vi "Plot.vi"(4 "Response Inverted?":bool, 6 "Stimulus Inverted?":bool, 8 "error in (no error)":errorcluster, 10 "Graph Manager.lvclass":refnum<class "Graph Manager.lvclass">, 11 "Sinusoidal Fit in":refnum<class "Abstract Fit.lvclass">) -> (0 "error out":errorcluster, 1 "Channel IDs":i32[](array[numeric]), 2 "Graph Manager.lvclass 2":refnum<class "Graph Manager.lvclass">, 3 "Sinusoidal Fit out":refnum<class "Abstract Fit.lvclass">)   [LabVIEW 2016, in "Abstract Fit.lvclass"]
uses:
  Abstract Fit.lvclass
  Graph Manager/Graph Manager.lvclass
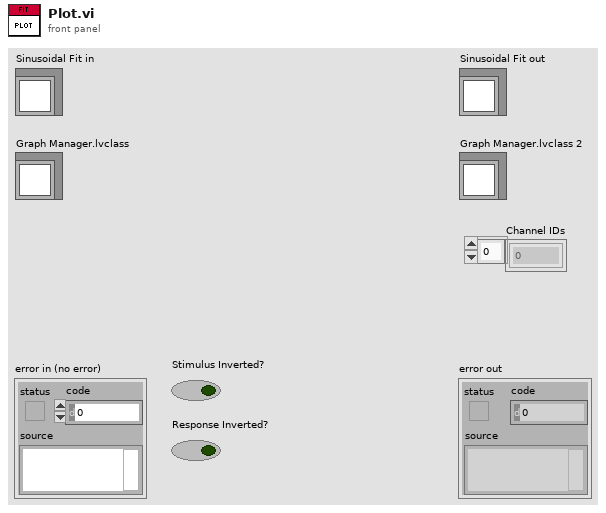
[diagram p1: front panel]
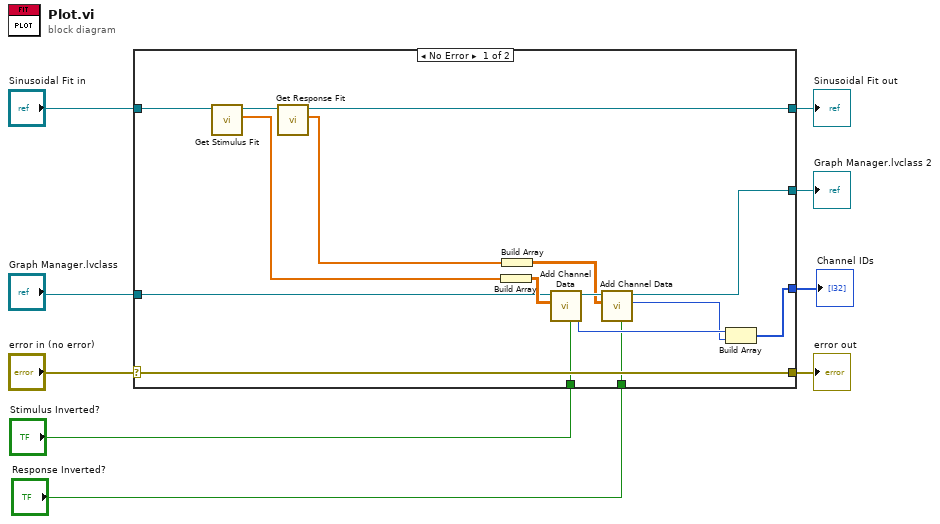
[diagram p0: block diagram]
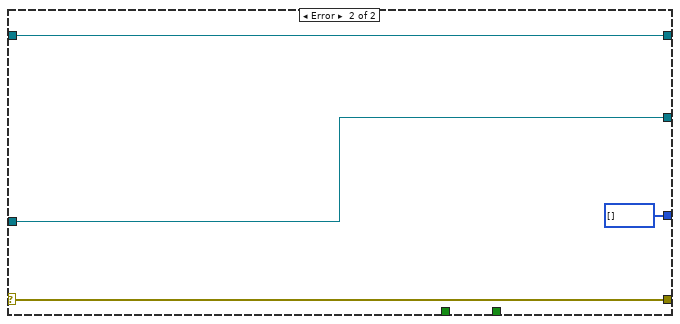
[diagram p2: hidden frame]
diagram:
  n1 = case shown="No Error" "error in (no error)" {
    selector: "error in (no error)" -> [w25 w29]
    tunnel: [w25 w29] -> w8
    tunnel: [w21 w28] -> w6
    tunnel: "Sinusoidal Fit in" -> [w23 w28]
    tunnel: "Graph Manager.lvclass" -> [w19 w27]
    tunnel: [w15 w27] -> w4
    tunnel: [w17 i32[] []] -> w3
    tunnel: "Stimulus Inverted?" -> [w11 _]
    tunnel: "Response Inverted?" -> [w10 _]
    frame No Error {
      n2 = call-dynamic "Get Stimulus Fit.vi"("Abstract Fit in"=w23) -> ("Fit out"=w20:dbl[], "Abstract Fit out"=w22:refnum<class "Abstract Fit.lvclass">)  [unwired: 8 in, 1 out]
      n3 = call-dynamic "Get Response Fit.vi"("Abstract Fit in"=w22) -> ("Fit out"=w14:dbl[], "Abstract Fit out"=w21:refnum<class "Abstract Fit.lvclass">)  [unwired: 8 in, 1 out]
      n4 = Build Array(w20) -> (w24:dbl[][])
      n5 = Build Array(w14) -> (w13:dbl[][])
      n6 = call-dynamic "Add Channel Data.vi"("Inverted?"=w11, "Channel Data"=w24, "Graph Manager in"=w19) -> ("Channel ID"=w18:i32, "Graph Manager out"=w16:refnum<class "Graph Manager.lvclass">)  [unwired: 6 in, 1 out]
      n7 = call-dynamic "Add Channel Data.vi"("Inverted?"=w10, "Channel Data"=w13, "Graph Manager in"=w16) -> ("Channel ID"=w12:i32, "Graph Manager out"=w15:refnum<class "Graph Manager.lvclass">)  [unwired: 6 in, 1 out]
      n8 = Build Array(w18, w12) -> (w17:i32[])
    }
    frame Error {
    }
  }
  "error out" <- w8
  "Sinusoidal Fit out" <- w6
  "Graph Manager.lvclass 2" <- w4
  "Channel IDs" <- w3
